vi "device_slots_positions.vi"(8 "error in":errorcluster, 11 "Sistema":refnum<k21>="localhost" caption="Session in") -> (0 "error out":errorcluster)   [LabVIEW 2018]
uses:
  config_board.ctl
  <vilib>/nisyscfg/nisyscfg.lvlib
  <resource>/objmgr/nisysapi.rc
panel:
  out "adress":string
  out "data":T1[](array[typedef])
  # "Aguarde enquanto o sistema é scaneado"
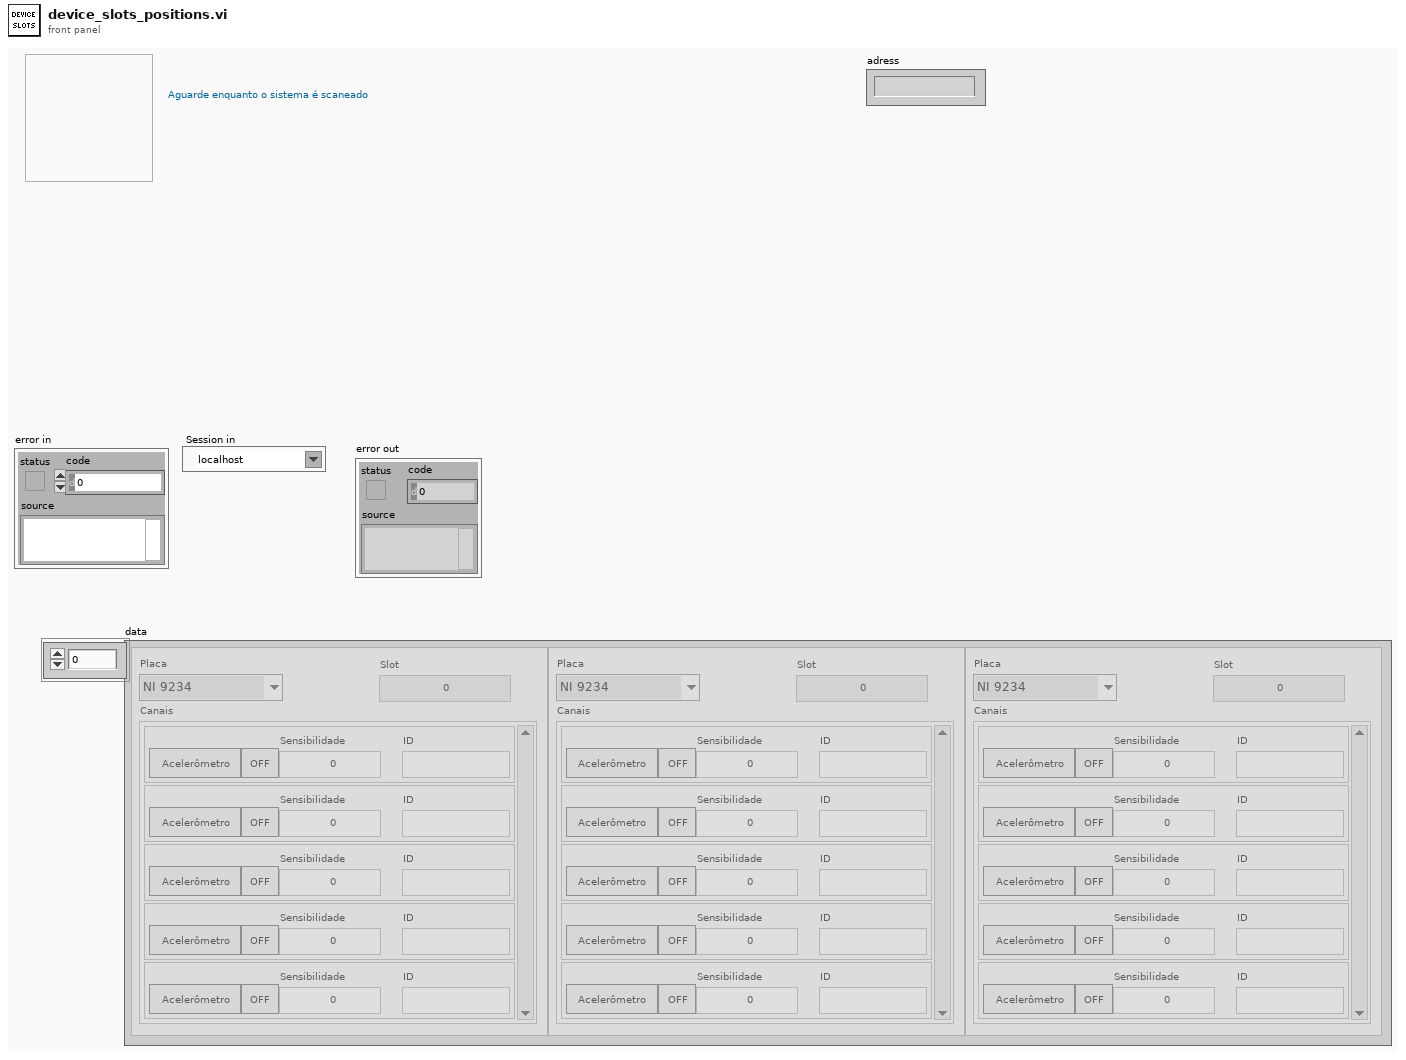
[diagram p1: front panel]
types:
  T1 = typedef "config_board.ctl" = cluster{"board":enum16{"NI 9234", "NI 9205", "Não aplicável"}, "channels":cluster{"type":bool, "active":bool, "sens":dbl, "ID":string}[], "Slot":i32}
  T2 = cluster{"type":bool, "active":bool, "Sens 4":i32, "ID":string}
  T3 = cluster{"type":bool, "active":bool, "Sens 4":dbl, "ID":string}[]
  T4 = cluster{"type":bool, "active":bool, "sens":dbl, "ID":string}[]
  T5 = cluster{"type":bool, "active":bool, "Sens 4":i32, "ID":string}[]
  T6 = cluster{"type":bool, "active":bool, "sens":dbl, "ID":string}
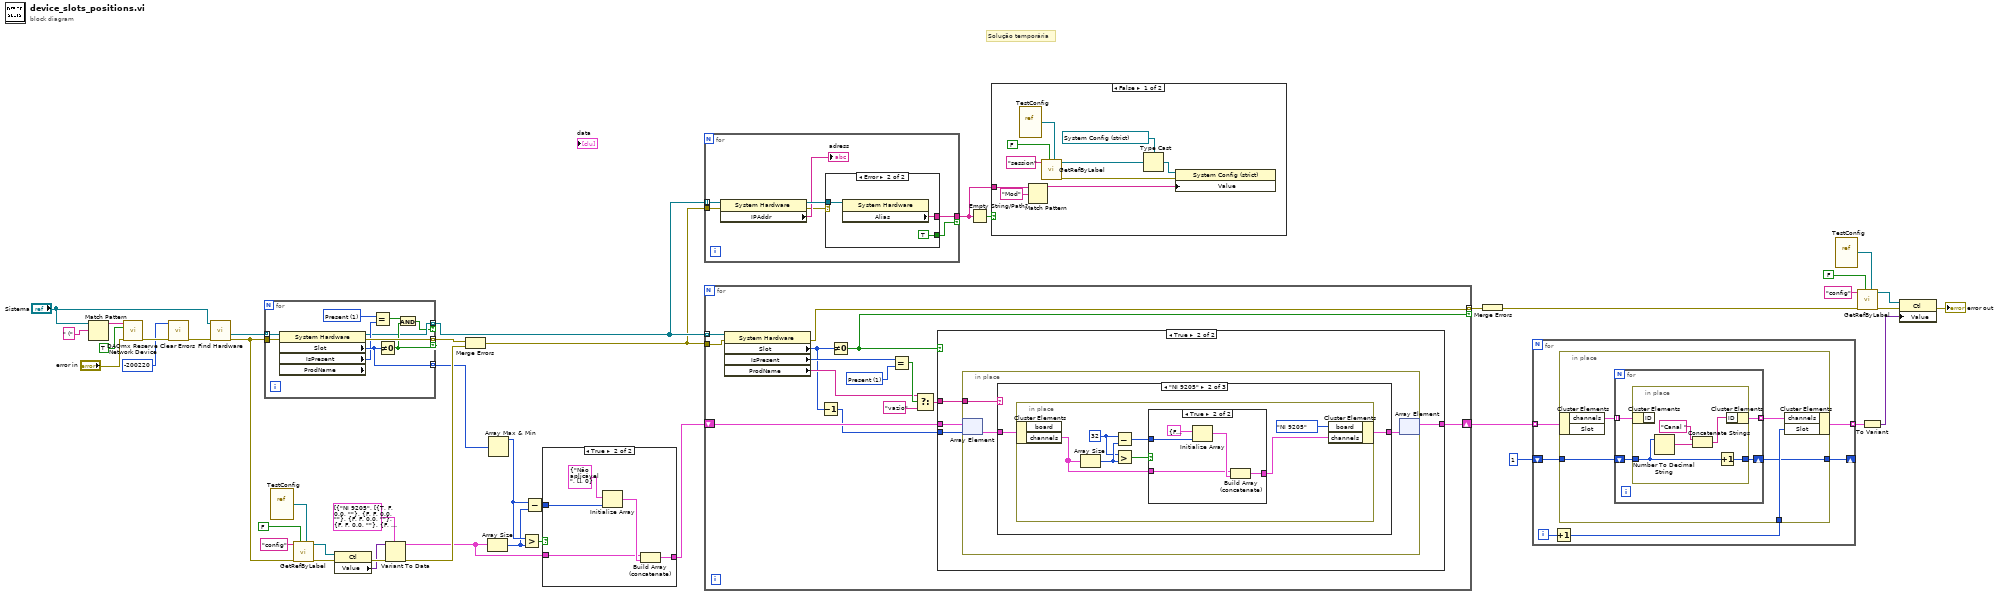
[diagram p0: block diagram]
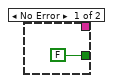
[diagram p3: hidden frame]
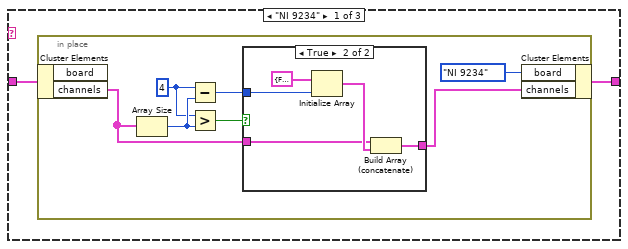
[diagram p5: hidden frame]
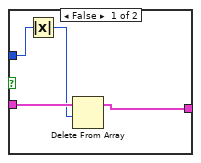
[diagram p6: hidden frame]
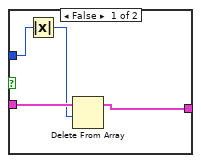
[diagram p7: hidden frame]
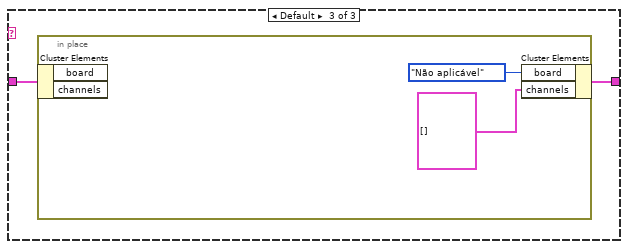
[diagram p8: hidden frame]
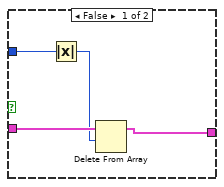
[diagram p9: hidden frame]
diagram:
  # "Solução temporária"
  n1 = Match Pattern(string="Sistema", regular expression=" (") -> (before substring=w11:string)  [unwired: 1 in, 3 out]
  n2 = call <vilib>:"DAQmx Reserve Network Device.vi"("device in"=w11, "override reservation?"=TRUE, "error in"="error in") -> ("error out"=w7:errorcluster)  [unwired: 11 in, 1 out]
  n3 = call <vilib>:"Clear Errors.vi"("error in (no error)"=w7, "specific error code to clear (0: all)"=-200220) -> ("error out"=w6:errorcluster)  [unwired: 4 in, 1 out]
  n4 = call <vilib>:"Find Hardware.vi"("error in (no error)"=w6, "Session in"="Sistema") -> ("error out"=w40:errorcluster, "Resources out"=w27:refnum<k20>[])  [unwired: 6 in, 2 out]
  n5 = for {
    tunnel: w27 -> [w53] mode=indexing
    tunnel: [w52] -> w26 mode=indexing if=w46
    tunnel: w40 -> [w51]
    tunnel: [w50] -> w34 mode=indexing
    tunnel: [w45] -> w4 mode=indexing if=w44
    w49 = 1 items=["Initializing"=-2, "Unknown"=-1, "Not Present"=0, "Present"=1] ("Devices & Chassis:Is Present")
    n6 = property class="System Hardware" props=["Slot", "IsPresent", "ProdName"](reference=w53, error in=w51) -> (reference out=w45:refnum<k20>, error out=w52:errorcluster, "Slot"=w50:i32, "IsPresent"=w48:i32)  [unwired: 1 out]
    n7 = Equal?(x=w49, y=w48) -> (x = y?=w47:bool)
    n8 = Not Equal To 0?(x=w50) -> (x != 0?=w46:bool)
    n9 = And(x=w47, y=w46) -> (x .and. y?=w44:bool)
  }
  n10 = vi-ref "TestConfig.vi"() -> (w41:refnum<vi>)
  n11 = call "GetRefByLabel.vi"("refVI"=w41, "InsideTab"=FALSE, "error in"=w40, "Label"="config") -> ("error out"=w39:errorcluster, "Ctl Refnum"=w38:refnum<vi>)  [unwired: 5 in, 1 out]
  n12 = property class="Ctl"(reference=w38, error in=w39) -> (error out=w37:errorcluster, "Value"=w36:variant)  [unwired: 1 out]
  n13 = Variant To Data(error in=w37, type=T1[] [{"board"=enum."NI 9205", "channels"=[{"type"=TRUE, "active"=FALSE, "sens"=0.0, "ID"=""}, {"type"=FALSE, "active"=FALSE, "sens"=0.0, "ID"=""}, {"type"=FALSE, "active"=FALSE, "sens"=0.0, "ID"=""}, {"type"=FALSE, "active"=FALSE, "sens"=0.0, "ID"=""}, {"type"=FALSE, "active"=FALSE, "sens"=0.0, "ID"=""}], "Slot"=0}, {"board"=enum."NI 9205", "channels"=[], "Slot"=0}] ("config"), Variant=w36) -> (data=w31:T1[], error out=w43:errorcluster)
  n14 = Merge Errors(w26, w43) -> (w3:errorcluster)
  n15 = Array Size(array=w31) -> (size(s)=w29:i32)
  n16 = Array Max & Min(array=w34) -> (max value=w30:i32)  [unwired: 3 out]
  n17 = Greater?(x=w30, y=w29) -> (0:w32:bool)
  n18 = Subtract(x=w30, y=w29) -> (x-y=w28:i32)
  n19 = case shown="True" w32 {
    tunnel: w31 -> [w56 w60]
    tunnel: w28 -> [w57 w59]
    tunnel: [w54 w58] -> w25
    frame False {
      n20 = Absolute Value(x=w57) -> (abs(x)=w55:i32)
      n21 = Delete From Array(array=w56, length=w55) -> (array with subset deleted=w54:T1[])  [unwired: 1 in, 1 out]
    }
    frame True {
      n22 = Initialize Array(T1 {"board"=enum."Não aplicável", "channels"=[], "Slot"=0} ("config_board"), w59) -> (w61:T1[])
      n23 = Build Array (concatenate)(w60, w61) -> (w58:T1[])
    }
  }
  n24 = for {
    tunnel: w4 -> [w69] mode=indexing
    tunnel: [w67] -> w1 if=w65
    tunnel: w3 -> [w64]
    n25 = property class="System Hardware"(reference=w69, error in=w64) -> (reference out=w68:refnum<k20>, error out=w63:errorcluster, "IPAddr"=→"adress":string)
    n26 = case shown="Error" w63 {
      tunnel: w68 -> [_ w73]
      tunnel: [_ w72] -> w67
      tunnel: [FALSE TRUE] -> w65
      frame No Error {
      }
      frame Error {
        n27 = property class="System Hardware"(reference=w73) -> ("Alias"=w72:string)  [unwired: 1 in, 2 out]
      }
    }
  }
  n28 = for {
    tunnel: w4 -> [w87] mode=indexing
    tunnel: w3 -> [w86]
    shift-right: [w76] -> w24
    shift-left: w25 -> [w80]
    tunnel: [w75] -> w17 mode=indexing if=w74
    w84 = 1 items=["Initializing"=-2, "Unknown"=-1, "Not Present"=0, "Present"=1] ("Devices & Chassis:Is Present")
    n29 = property class="System Hardware"(reference=w87, error in=w86) -> (error out=w75:errorcluster, "Slot"=w79:i32, "IsPresent"=w85:i32, "ProdName"=w82:string)  [unwired: 1 out]
    n30 = Decrement(x=w79) -> (x-1=w78:i32)
    n31 = Not Equal To 0?(x=w79) -> (x != 0?=w74:bool)
    n32 = Equal?(x=w85, y=w84) -> (x = y?=w83:bool)
    n33 = Select(t=w82, s=w83, f="vazio") -> (s? t:f=w77:string)
    n34 = case shown="True" w74 {
      tunnel: w80 -> [w88 w92]
      tunnel: w78 -> [_ w91]
      tunnel: w77 -> [_ w90]
      tunnel: [w88 w89] -> w76
      frame False {
      }
      frame True {
        n35 = in-place {
          in-place-border: w90 -> [w95]
          n36 = in-place-array #1(w92, w91) -> (w94:T1)
          n37 = case shown="\"NI 9205\"" w95 {
            tunnel: w94 -> [w97 w115 w133]
            tunnel: [w96 w114 w132] -> w93
            frame "NI 9234" {
              n38 = in-place {
                w99 = 4 ("size(s)")
                n39 = in-place-cluster #2(w97) -> ("channels"=w100:T4)  [unwired: 1 out]
                n40 = Array Size(array=w100) -> (size(s)=w102:i32)
                n41 = Subtract(x=w99, y=w102) -> (x-y=w101:i32)
                n42 = Greater?(x=w99, y=w102) -> (0:w103:bool)
                n43 = case shown="True" w103 {
                  tunnel: w100 -> [w107 w112]
                  tunnel: w101 -> [w108 w111]
                  tunnel: [w105 w110] -> w98
                  frame False {
                    n44 = Absolute Value(x=w108) -> (abs(x)=w106:i32)
                    n45 = Delete From Array(array=w107, length=w106) -> (array with subset deleted=w105:T4)  [unwired: 1 in, 1 out]
                  }
                  frame True {
                    n46 = Initialize Array(T2 {"type"=FALSE, "active"=FALSE, "Sens 4"=1, "ID"=""} ("config"), w111) -> (w113:T5)
                    n47 = Build Array (concatenate)(w112, w113) -> (w110:T4)
                  }
                }
                n48 = in-place-cluster #2("board"=enum16{"NI 9234", "NI 9205", "Não aplicável"}."NI 9234", "channels"=w98) -> (w96:T1)
              }
            }
            frame "NI 9205" {
              n49 = in-place {
                w117 = 32 ("size(s)")
                n50 = in-place-cluster #3(w115) -> ("channels"=w118:T4)  [unwired: 1 out]
                n51 = Array Size(array=w118) -> (size(s)=w120:i32)
                n52 = Subtract(x=w117, y=w120) -> (x-y=w119:i32)
                n53 = Greater?(x=w117, y=w120) -> (0:w121:bool)
                n54 = case shown="True" w121 {
                  tunnel: w118 -> [w125 w130]
                  tunnel: w119 -> [w126 w129]
                  tunnel: [w123 w128] -> w116
                  frame False {
                    n55 = Absolute Value(x=w126) -> (abs(x)=w124:i32)
                    n56 = Delete From Array(array=w125, length=w124) -> (array with subset deleted=w123:T4)  [unwired: 1 in, 1 out]
                  }
                  frame True {
                    n57 = Initialize Array(T2 {"type"=FALSE, "active"=FALSE, "Sens 4"=1, "ID"=""} ("config"), w129) -> (w131:T5)
                    n58 = Build Array (concatenate)(w130, w131) -> (w128:T4)
                  }
                }
                n59 = in-place-cluster #3("board"=enum16{"NI 9234", "NI 9205", "Não aplicável"}."NI 9205", "channels"=w116) -> (w114:T1)
              }
            }
            frame Default {
              n60 = in-place {
                n61 = in-place-cluster #4(w133) -> ()  [unwired: 2 out]
                n62 = in-place-cluster #4("board"=enum16{"NI 9234", "NI 9205", "Não aplicável"}."Não aplicável", "channels"=T3 []) -> (w132:T1)
              }
            }
          }
          n63 = in-place-array #1(w93) -> (w89:T1[])  [unwired: 1 out]
        }
      }
    }
  }
  n64 = Empty String/Path?(string/path=w1) -> (empty?=w2:bool)
  n65 = case shown="False" w2 {
    tunnel: w1 -> [w145 _]
    frame False {
      n66 = vi-ref "TestConfig.vi"() -> (w142:refnum<vi>)
      n67 = Match Pattern(string=w145, regular expression="Mod") -> (before substring=w136:string)  [unwired: 1 in, 3 out]
      n68 = call "GetRefByLabel.vi"("refVI"=w142, "InsideTab"=FALSE, "Label"="session") -> ("error out"=w141:errorcluster, "Ctl Refnum"=w139:refnum<vi>)  [unwired: 6 in, 1 out]
      n69 = Type Cast(type=refnum<vi> refnum ("session"), x=w139) -> (*(type *) &x=w137:refnum<vi>)
      n70 = property class="System Config (strict)"(reference=w137, error in=w141, "Value"=w136) -> ()  [unwired: 2 out]
    }
    frame True {
    }
  }
  n71 = Merge Errors(w17) -> (w16:errorcluster)
  n72 = for {
    tunnel: w24 -> [w151] mode=indexing
    shift-right: [w147] -> _
    shift-left: 1 -> [w148]
    tunnel: [w146] -> w15 mode=indexing
    i -> [w150]
    n73 = Increment(x=w150) -> (x+1=w149:i32)
    n74 = in-place {
      in-place-border: w149 -> [w156]
      in-place-border: w148 -> [w154]
      in-place-border: [w153] -> w147
      n75 = in-place-cluster #5(w151) -> ("channels"=w155:T4)  [unwired: 1 out]
      n76 = for {
        tunnel: w155 -> [w160] mode=indexing
        shift-right: [w158] -> w153
        shift-left: w154 -> [w159]
        tunnel: [w157] -> w152 mode=indexing
        n77 = in-place {
          in-place-border: w159 -> [w164]
          in-place-border: [w165] -> w158
          n78 = in-place-cluster #6(w160) -> ()  [unwired: 1 out]
          n79 = Number To Decimal String(number=w164) -> (decimal integer string=w163:string)  [unwired: 1 in]
          n80 = Concatenate Strings("Canal " ("string"), w163) -> (w161:string)
          n81 = Increment(x=w164) -> (x+1=w165:i32)
          n82 = in-place-cluster #6("ID"=w161) -> (w157:T6)
        }
      }
      n83 = in-place-cluster #5("channels"=w152, "Slot"=w156) -> (w146:T1)
    }
  }
  n84 = vi-ref "TestConfig.vi"() -> (w21:refnum<vi>)
  n85 = call "GetRefByLabel.vi"("refVI"=w21, "InsideTab"=FALSE, "error in"=w16, "Label"="config") -> ("error out"=w20:errorcluster, "Ctl Refnum"=w19:refnum<vi>)  [unwired: 5 in, 1 out]
  n86 = To Variant(anything=w15) -> (Variant=w14:variant)
  n87 = property class="Ctl"(reference=w19, error in=w20, "Value"=w14) -> (error out=→"error out":errorcluster)  [unwired: 1 out]
